vi "EnFlo_Lab_Temp_Control.vi"(0 "EnFlo Lab:Heat:Extraction":dbl format="%.2f") -> ()   [LabVIEW 2015]
uses:
  ADAM Client/Sub VIs/ADAM Controls/Update_scan_value.ctl
panel:
  out "EnFlo Lab:labstrat1:Av Temp":dbl
  out "EnFlo_Tunnel:Exit Duct:Dem Temp":dbl
  out "Reduction in air temp from ambient":dbl
  out "Approx Heat Extraction Value in kW":dbl
  out "EnFlo Lab:Desired:Air Temp":dbl
  out "Temperature Error":dbl
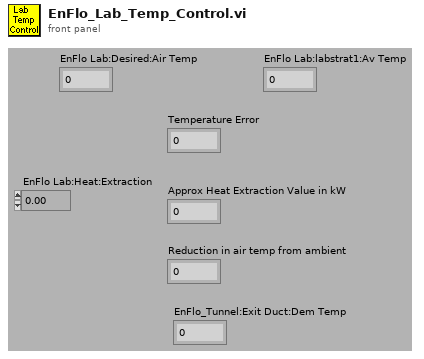
[diagram p1: front panel]
types:
  T1 = enum16{"Append to Global", "Read Global then Clear"}
  T2 = typedef "Update_scan_value.ctl" = cluster{"Channel Name":string, "New Value":dbl}
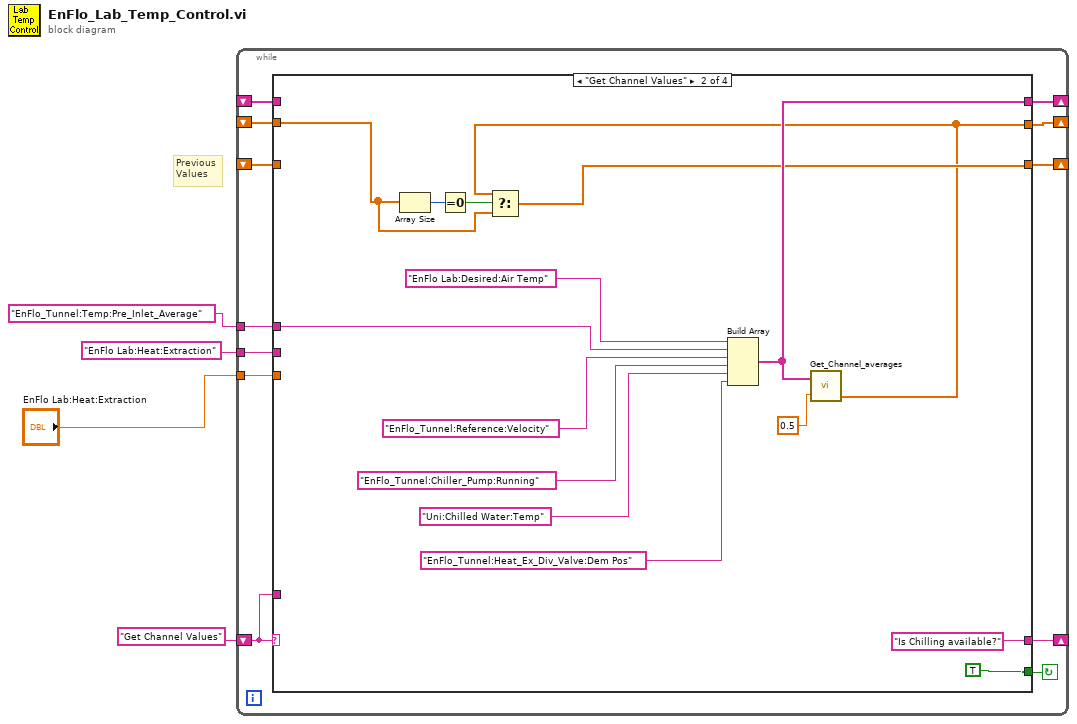
[diagram p0: block diagram]
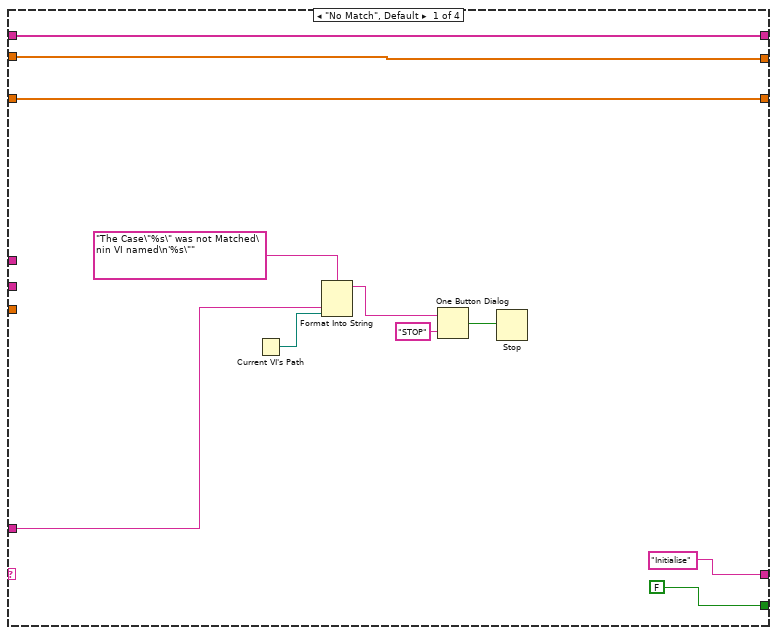
[diagram p2: hidden frame]
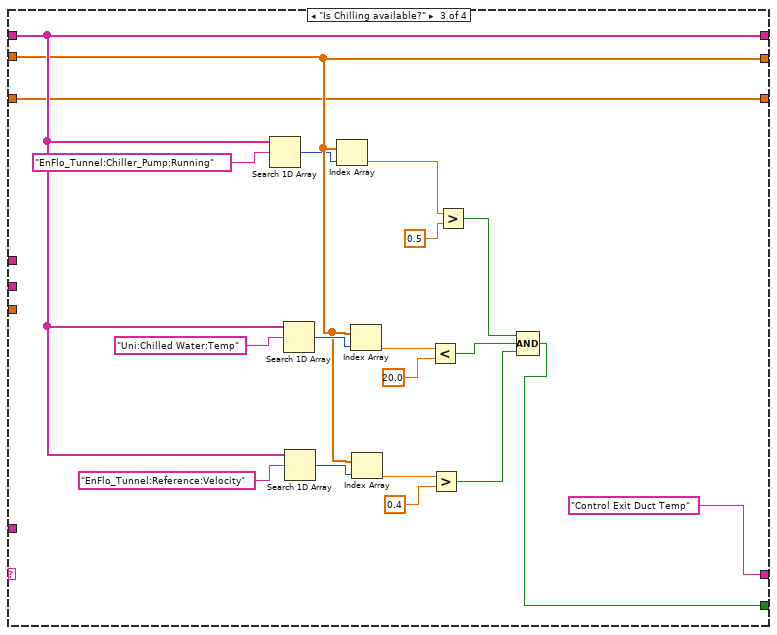
[diagram p3: hidden frame]
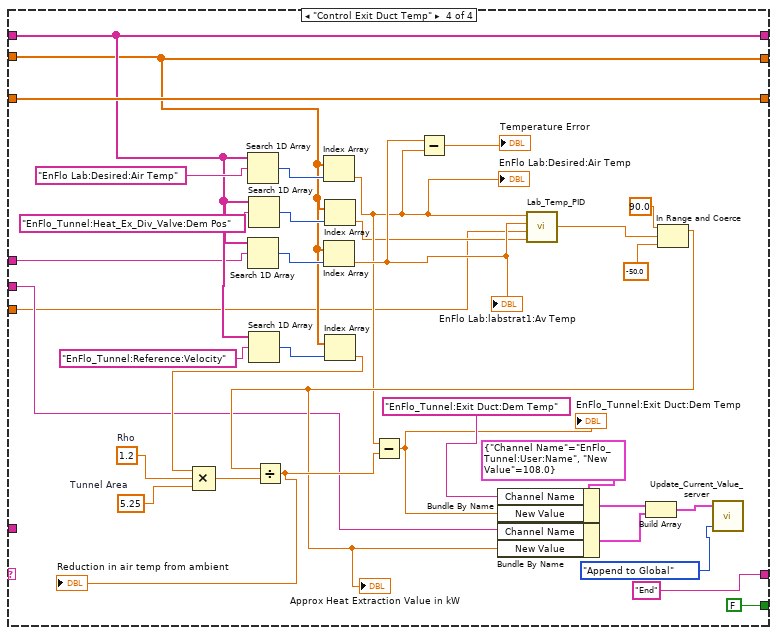
[diagram p4: hidden frame]
diagram:
  # "Previous\nValues"
  n1 = while {
    shift-left: "Get Channel Values" -> [w14]
    shift-right: [w15] -> _
    shift-right: [w12] -> _
    shift-left: _ -> [w10]
    shift-right: [w13] -> _
    shift-left: _ -> [w11]
    shift-right: [w9] -> _
    shift-left: _ -> [w8]
    tunnel: "EnFlo Lab:Heat:Extraction" -> [w7]
    tunnel: "EnFlo Lab:Heat:Extraction" -> [w6]
    tunnel: "EnFlo_Tunnel:Temp:Pre_Inlet_Average" -> [w5]
    stop <- w16 continue-if-true
    n2 = case shown="\"Get Channel Values\"" w14 {
      tunnel: [FALSE TRUE w43 FALSE] -> w16
      tunnel: ["Initialise" "Is Chilling available?" "Control Exit Duct Temp" "End"] -> w15
      tunnel: w14 -> [w22 _ _ _]
      tunnel: [w19 w29 w49 w67] -> w13
      tunnel: [w18 w36 w50 w69] -> w12
      tunnel: w11 -> [w19 w30 w49 w67]
      tunnel: w10 -> [w18 _ w50 w69]
      tunnel: [w17 w31 w48 w90] -> w9
      tunnel: w8 -> [w17 _ w48 w90]
      tunnel: w7 -> [_ _ _ w65]
      tunnel: w6 -> [_ _ _ w64]
      tunnel: w5 -> [_ w28 _ w63]
      frame "No Match", Default {
        n3 = Current VI's Path() -> (path=w21:path)
        n4 = Format Into String(format string="The Case\"%s\" was not Matched\nin VI named\n'%s\"" ("Format String"), w22, w21) -> (resulting string=w25:string)  [unwired: 2 in, 1 out]
        n5 = One Button Dialog(message=w25, button name ("OK")="STOP") -> (true=w23:bool)
        n6 = Stop(stop? (T)=w23) -> ()
      }
      frame "Get Channel Values" {
        n7 = Array Size(array=w30) -> (size(s)=w33:i32)
        n8 = Equal To 0?(x=w33) -> (x = 0?=w32:bool)
        n9 = Build Array("EnFlo Lab:Desired:Air Temp", w28, "EnFlo_Tunnel:Reference:Velocity", "EnFlo_Tunnel:Chiller_Pump:Running", "Uni:Chilled Water:Temp", "EnFlo_Tunnel:Heat_Ex_Div_Valve:Dem Pos") -> (w36:string[])
        n10 = call "Get_Channel_averages.vi"("Desired Ch Names"=w36, "Averaging time (mins)"=0.5) -> ("number"=w29:dbl[])  [unwired: 1 in, 2 out]
        n11 = Select(t=w29, s=w32, f=w30) -> (s? t:f=w31:dbl[])
      }
      frame "Is Chilling available?" {
        n12 = Search 1D Array(1D array=w50, element="EnFlo_Tunnel:Chiller_Pump:Running") -> (index of element=w47:i32)  [unwired: 1 out]
        n13 = Search 1D Array(1D array=w50, element="Uni:Chilled Water:Temp") -> (index of element=w60:i32)  [unwired: 1 out]
        n14 = Search 1D Array(1D array=w50, element="EnFlo_Tunnel:Reference:Velocity") -> (index of element=w55:i32)  [unwired: 1 out]
        n15 = Index Array(array=w49, index=w47) -> (element=w44:dbl)
        n16 = Index Array(array=w49, index=w60) -> (element=w59:dbl)
        n17 = Index Array(array=w49, index=w55) -> (element=w56:dbl)
        n18 = Less?(x=w59, y=20.0) -> (x < y?=w53:bool)
        n19 = Greater?(x=w56, y=0.4) -> (0:w52:bool)
        n20 = Greater?(x=w44, y=0.5) -> (0:w45:bool)
        n21 = Compound Arithmetic op=AND(w45, w53, w52) -> (w43:bool)
      }
      frame "Control Exit Duct Temp" {
        w75 = T2 {"Channel Name"="EnFlo_Tunnel:User:Name", "New Value"=108.0} ("Update Scan Value Cluster")
        w87 = 5.25  # Tunnel Area
        w88 = 1.2  # Rho
        n22 = Search 1D Array(1D array=w69, element="EnFlo Lab:Desired:Air Temp") -> (index of element=w97:i32)  [unwired: 1 out]
        n23 = Search 1D Array(1D array=w69, element=w63) -> (index of element=w94:i32)  [unwired: 1 out]
        n24 = Search 1D Array(1D array=w69, element="EnFlo_Tunnel:Heat_Ex_Div_Valve:Dem Pos") -> (index of element=w70:i32)  [unwired: 1 out]
        n25 = Search 1D Array(1D array=w69, element="EnFlo_Tunnel:Reference:Velocity") -> (index of element=w91:i32)  [unwired: 1 out]
        n26 = Index Array(array=w67, index=w97) -> (element=w71:dbl)
        "EnFlo Lab:Desired:Air Temp" <- w71
        n27 = Index Array(array=w67, index=w94) -> (element=w73:dbl)
        "EnFlo Lab:labstrat1:Av Temp" <- w73
        n28 = Index Array(array=w67, index=w70) -> (element=w66:dbl)
        n29 = Index Array(array=w67, index=w91) -> (element=w89:dbl)
        n30 = Compound Arithmetic op=MULTIPLY(w89, w88, w87) -> (w86:dbl)
        n31 = Subtract(x=w73, y=w71) -> (x-y=→"Temperature Error":dbl)
        n32 = call "Lab_Temp_PID.vi"("Valve Pos"=w66, "Previous Control Sum"=w64, "Present Value"=w73, "Setpoint"=w71) -> ("Dem Output"=w74:dbl)
        n33 = In Range and Coerce(upper limit=90.0, x=w74, lower limit=-50.0) -> (coerced(x)=w77:dbl)  [unwired: 1 out]
        "Approx Heat Extraction Value in kW" <- w77
        n34 = Divide(x=w77, y=w86) -> (x/y=w85:dbl)
        "Reduction in air temp from ambient" <- w85
        n35 = Subtract(x=w71, y=w85) -> (x-y=w81:dbl)
        "EnFlo_Tunnel:Exit Duct:Dem Temp" <- w81
        n36 = Bundle By Name(cluster=w75, "Channel Name"="EnFlo_Tunnel:Exit Duct:Dem Temp", "New Value"=w81) -> (w78:T2)
        n37 = Bundle By Name(cluster=w75, "Channel Name"=w65, "New Value"=w77) -> (w76:T2)
        n38 = Build Array(w78, w76) -> (w83:T2[])
        n39 = call "Update_Current_Value_server.vi"("Mode"=T1."Append to Global", "Update array in"=w83) -> ()  [unwired: 1 in, 1 out]
      }
    }
  }
